vi "DDAQ-Open.vi"(8 "error in (no error)":errorcluster, 11 "IP Address of Nucleo Device":string="192.168.203.151") -> (0 "error out":errorcluster, 3 "connection ID":refnum<k5>, 4 "Elapsed time, ms (debug)":u32)   [LabVIEW 2020]
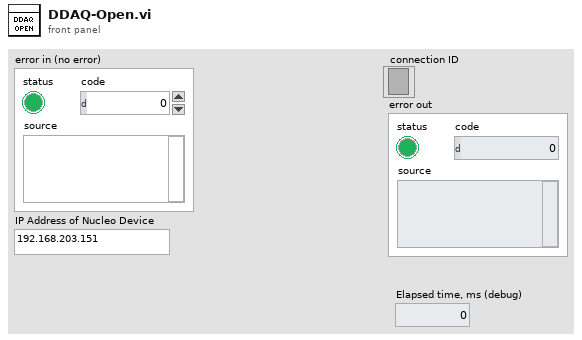
[diagram p1: front panel]
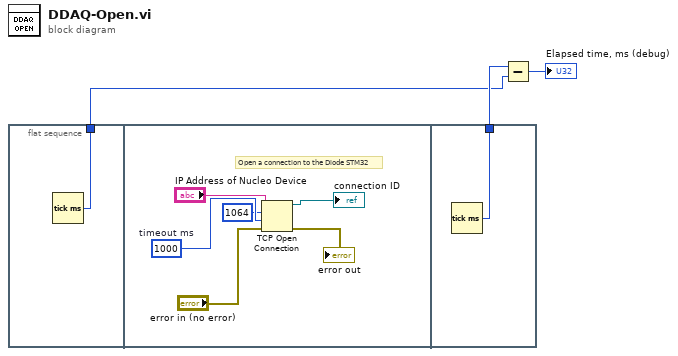
[diagram p0: block diagram]
diagram:
  n1 = flat-sequence {
    tunnel: [w4] -> w2
    tunnel: [w11] -> w3
    frame #0 {
      n2 = Tick Count (ms)() -> (millisecond timer value=w4:u32)
    }
    frame #1 {
      w6 = 1000  # timeout ms
      # "Open a connection to the Diode STM32"
      n3 = TCP Open Connection(address="IP Address of Nucleo Device", remote port or service name=u16 1064, timeout ms (60000)=w6, error in (no error)="error in (no error)") -> (connection ID=→"connection ID":refnum<k5>, error out=→"error out":errorcluster)  [unwired: 1 in]
    }
    frame #2 {
      n4 = Tick Count (ms)() -> (millisecond timer value=w11:u32)
    }
  }
  n5 = Subtract(x=w3, y=w2) -> (x-y=→"Elapsed time, ms (debug)":u32)
